vi "CTRE_CANTalonSRX_UpdateRefNum.vi"(10 "Update":bool, 11 "CAN Talon SRX Ref":T1={"DeviceStatus"={"status"=FALSE, "code"=0, "source"=""}, "Type"=enum."PWM", "PWM"={"PWM Channel"=enum."Invalid", "DeadBand"={"Name"="", "maxPositivePwm"=0, "minPositivePwm"=0, "centerPwm"=0, "maxNegativePwm"=0, "minNegativePwm"=0, "angularRange"=0}}, "CAN"={"Device Number"=0, "SetOutput VI Ref"=variant, "GetOutput VI Ref"=variant, "Enable VI Ref"=variant, "Disable VI Ref"=variant, "Data"=variant}, "Invert"=FALSE}) -> (3 "CAN Talon SRX Ref":T1={"DeviceStatus"={"status"=FALSE, "code"=0, "source"=""}, "Type"=enum."PWM", "PWM"={"PWM Channel"=enum."Invalid", "DeadBand"={"Name"="", "maxPositivePwm"=0, "minPositivePwm"=0, "centerPwm"=0, "maxNegativePwm"=0, "minNegativePwm"=0, "angularRange"=0}}, "CAN"={"Device Number"=0, "SetOutput VI Ref"=variant, "GetOutput VI Ref"=variant, "Enable VI Ref"=variant, "Disable VI Ref"=variant, "Data"=variant}, "Invert"=FALSE})   [LabVIEW 2016]
uses:
  <vilib>/Rock Robotics/WPI/MotorControl/WPI_MotorControlDeviceRef.ctl
  <vilib>/Rock Robotics/WPI/MotorControl/WPI_MotorControlType.ctl
  <vilib>/Rock Robotics/SystemInterfaces/DIO/FPGA_DIOPWMChannel.ctl
  <vilib>/Rock Robotics/WPI/PWM/WPI_PWMDeadband.ctl
  <vilib>/Rock Robotics/WPI/ThirdParty/CanMotor/CTRLib-LV-TalonSRX/TalonSRXDevRefData.ctl
  <vilib>/Rock Robotics/WPI/ThirdParty/CanMotor/CTRLib-LV-TalonSRX/CTRE_CANTalonSRX_ControlMode.ctl
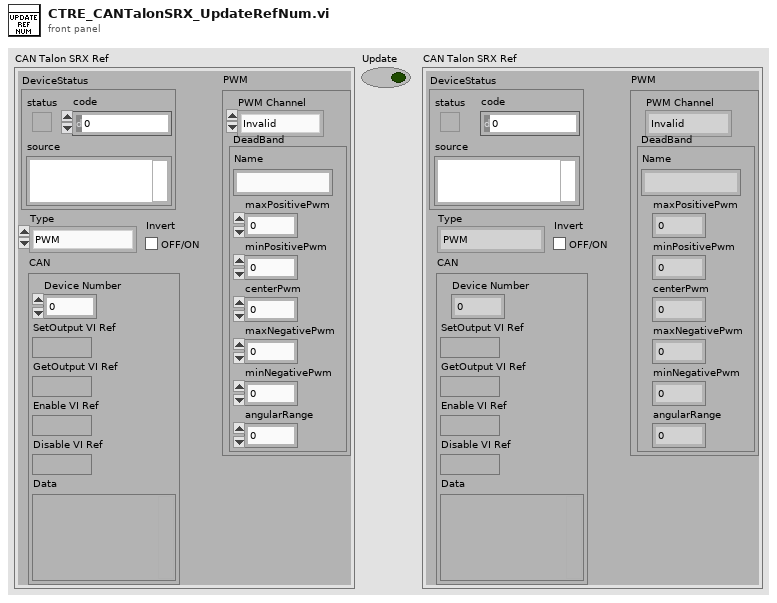
[diagram p1: front panel]
types:
  T1 = typedef "WPI_MotorControlDeviceRef.ctl" = cluster{"DeviceStatus":errorcluster, "Type":T2, "PWM":cluster{"PWM Channel":T3, "DeadBand":T4}, "CAN":cluster{"Device Number":u8, "SetOutput VI Ref":variant, "GetOutput VI Ref":variant, "Enable VI Ref":variant, "Disable VI Ref":variant, "Data":variant}, "Invert":bool}
  T2 = typedef "WPI_MotorControlType.ctl" = enum16{"PWM", "CAN"}
  T3 = typedef "FPGA_DIOPWMChannel.ctl" = enum8{"PWM 0", "PWM 1", "PWM 2", "PWM 3", "PWM 4", "PWM 5", "PWM 6", "PWM 7", "PWM 8", "PWM 9", "PWM MXP 0", "PWM MXP 1", "PWM MXP 2", "PWM MXP 3", "PWM MXP 4", "PWM MXP 5", "PWM MXP 6", "PWM MXP 7", "PWM MXP 8", "PWM MXP 9", "Invalid"}
  T4 = typedef "WPI_PWMDeadband.ctl" = cluster{"Name":string, "maxPositivePwm":i32, "minPositivePwm":i32, "centerPwm":i32, "maxNegativePwm":i32, "minNegativePwm":i32, "angularRange":u16}
  T5 = typedef "TalonSRXDevRefData.ctl" = cluster{"Library":path, "handle":u64, "Talon SRX Mode":T6, "UsageFrame":u32, "RefNumName":string}
  T6 = typedef "CTRE_CANTalonSRX_ControlMode.ctl" = enum16{"Throttle (Duty-Cycle)", "Position Closed-Loop", "Velocity Closed-Loop", "Current Closed-Loop", "Voltage Compensation", "Slave Follower", "Motion Profile", "Motion Magic"}
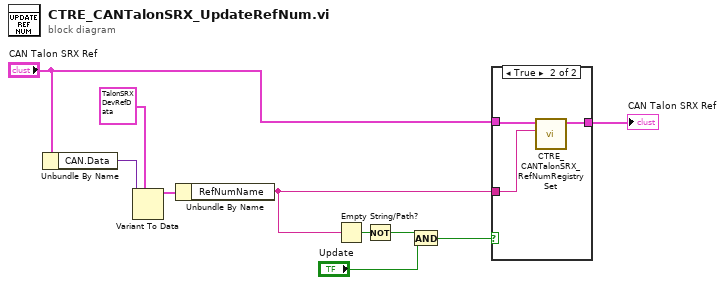
[diagram p0: block diagram]
diagram:
  n1 = Unbundle By Name("CAN Talon SRX Ref") -> ("CAN.Data"=w9:variant)
  n2 = Variant To Data(type=T5 {"Library"=path "", "handle"=0, "Talon SRX Mode"=enum."Throttle (Duty-Cycle)", "UsageFrame"=0, "RefNumName"=""}, Variant=w9) -> (data=w7:T5)  [unwired: 1 in, 1 out]
  n3 = Unbundle By Name(w7) -> ("RefNumName"=w2:string)
  n4 = Empty String/Path?(string/path=w2) -> (empty?=w6:bool)
  n5 = Not(x=w6) -> (.not. x?=w5:bool)
  n6 = And(x=w5, y="Update") -> (x .and. y?=w3:bool)
  n7 = case shown="True" w3 {
    tunnel: "CAN Talon SRX Ref" -> [w11 w13]
    tunnel: [w11 w14] -> w10
    tunnel: w2 -> [_ w12]
    frame False {
    }
    frame True {
      n8 = call <vilib>:"CTRE_CANTalonSRX_RefNumRegistrySet.vi"("refnum name"=w12, "MotorControlDevRef"=w13) -> ("MotorControlDevRef"=w14:T1)  [unwired: 9 in]
    }
  }
  "CAN Talon SRX Ref" <- w10
